vi "3.2.2.-Sistema HSV sin Formula Node.vi"() -> ()   [LabVIEW 2020]
panel:
  out "Color Box 2":u32(colorbox)
  out "H":dbl(knob) scale=0.0..1.0 scale format="%#_10g"
  out "V":dbl(slide) scale=0.0..1.0
  out "S":dbl(slide) scale=0.0..1.0
  in  "B":u8(slide) scale=0.0..255.0
  in  "G":u8(slide) scale=0.0..255.0
  in  "R":u8(slide) scale=0.0..255.0
  # "di_cer0 - Visión Artificial - LabVIEW"
  # "HSV: La variable V llamada valor empieza desde la base del cono de colores, yendo del color nego hacia el blanco que se encuentra en el centro del círculo superior del cono, es básicamente la altura en el cono de colores, haciendo referencias a los niveles de grises.\n- El color negro puro corresponde al valor de V = 0.\n- El valor de 0 < V < 1 ocupa todos los niveles de grises.\n- El color blanco puro corresponde al valor de V = 1."
  # "HSV: La variable H llamada matiz empieza en el color rojo y le da un giro completo a la esfera del cono de colores obtenido a partir del cubo de colores, yendo de 0 a 1.\n- Rojo puro corresponde al valor de H = 0 o H =1.\n- El color amarillo vale H = 1/6 = 0.16.\n- El verde vale H = 1/3 = 0.33.\n- El color cian (azul cielo) se encuentra a H = 1/2 = 0.5.\n- El color azul (azul rey) se encuentra a H = 2/3 = 0.66.\n- El magenta se encuentra en H = 5/6 = 0.83. \nEl matiz nunca alcanza al color blanco o negro."
  # "HSV: La variable S llamada saturación empieza del centro del círculo que va del color blanco hacia los extremos del círculo donde se encuentra H (matiz) yendo de 0 a 1.\n- El color blanco puro corresponde al valor de S = 0.\n- El valor de 0 < S < 1 lo que hace es hacer pálidos los matices de colores que se encuentran en el perímetro de la circunferencia.\n- El valor de S que muestra el rango de colores en su máxima expresión es S = 1, por lo que muestra colores puros."
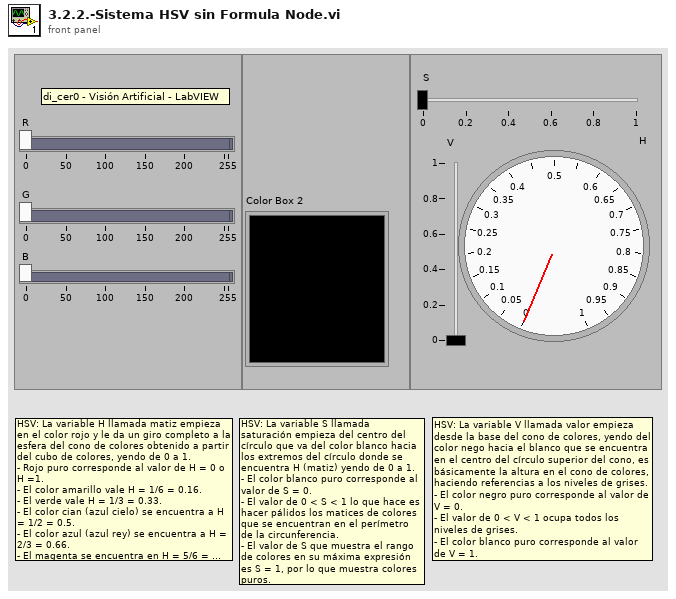
[diagram p1: front panel]
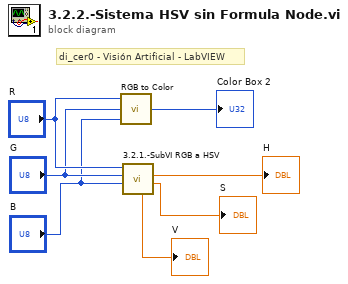
[diagram p0: block diagram]
diagram:
  # "di_cer0 - Visión Artificial - LabVIEW"
  n1 = call <vilib>:"RGB to Color.vi"("B"="B", "G"="G", "R"="R") -> ("Color"=→"Color Box 2":u32)
  n2 = call "3.2.1.-SubVI RGB a HSV.vi"("B"="B", "G"="G", "R"="R") -> ("S"=→"S":dbl, "V"=→"H":dbl, "H"=→"V":dbl)  [unwired: 6 in]
